vi "Secure-Release Region.vi"(7 "Action":enum16{"Secure", "Release"}(ring), 8 "error in (no error)":errorcluster, 10 "Control In":T1={"I-O.lvclass"=refnum, "Motion.lvclass"=refnum, "Dispenser.lvclass"=refnum}, 11 "Workspace in":refnum<class "Component Tray.lvclass">) -> (0 "error out":errorcluster, 2 "Control Out":T1, 3 "Workspace out":refnum<class "Component Tray.lvclass">)   [LabVIEW 2016, in "Component Tray.lvclass"]
uses:
  Component Tray.lvclass
  C:/Users/HEP Gantry/Documents/Assembly/V5/Classes/Workspace/Fixture.lvclass
  Controller/Controllers.ctl
  Controller/I-O/I-O.lvclass
  Controller/Motion/A3200/A3200.lvclass
  Controller/Dispenser/Dispenser.lvclass
  Controller/Motion/Motion.lvclass
  Fixture.lvclass/Fixture.ctl
  Read Gantry Region.vi
  Read Position.vi
  Fixture.lvclass
  Controller/Controller.lvclass
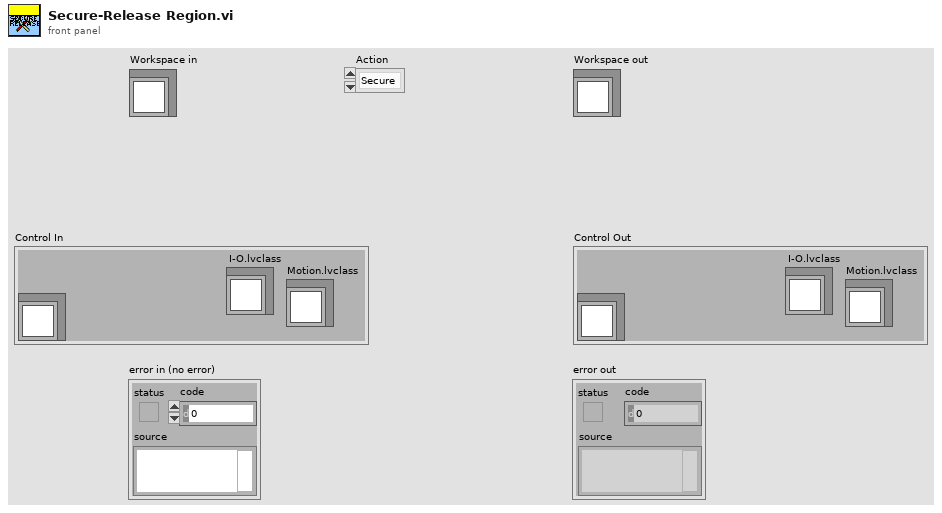
[diagram p1: front panel]
types:
  T1 = typedef "Controller.lvclass/Controllers.ctl" = cluster{"I-O.lvclass":refnum<class "I-O.lvclass">, "Motion.lvclass":refnum<class "Motion.lvclass">, "Dispenser.lvclass":refnum<class "Dispenser.lvclass">}
  T2 = typedef "I-O.lvclass/Pin Map.ctl" = cluster{"Region Valves":i32[], "Extra Valves":dbl[][], "Tool Primary Valve":i32, "Tool Secondary Valve":i32, "Region Sensors":i32[], "Extra Sensors":dbl[][], "Tool Primary Sensor":dbl, "Tool Secondary Sensor":dbl, "Compression Sensor":dbl, "5V":i32}
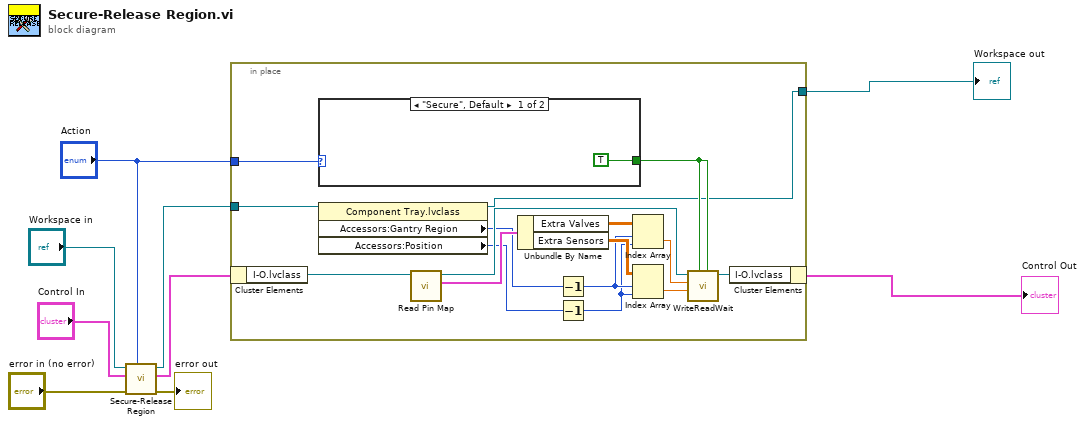
[diagram p0: block diagram]
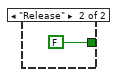
[diagram p2: hidden frame]
diagram:
  n1 = call-parent "Secure-Release Region.vi"("Action"="Action", "error in (no error)"="error in (no error)", "Control In"="Control In", "Fixture in"="Workspace in") -> ("error out"=→"error out":errorcluster, "Control Out"=w5:T1, "Fixture out"=w2:refnum<class "Component Tray.lvclass">)  [unwired: 5 in]
  n2 = in-place {
    in-place-border: "Action" -> [w22]
    in-place-border: w2 -> [w19]
    in-place-border: [w12] -> w1
    n3 = in-place-cluster #1(w5) -> ("I-O.lvclass"=w24:refnum<class "I-O.lvclass">)
    n4 = case shown="\"Secure\", Default" w22 {
      tunnel: [TRUE FALSE] -> w23
      frame "Secure", Default {
      }
      frame "Release" {
      }
    }
    n5 = property class="Component Tray.lvclass"(reference=w19) -> (reference out=w12:refnum<class "Component Tray.lvclass">, "Accessors:Gantry Region"=w16:i32, "Accessors:Position"=w14:i32)  [unwired: 1 in, 1 out]
    n6 = call-dynamic "Read Pin Map.vi"("I-O in"=w24) -> ("Pin Map"=w25:T2, "I-O out"=w21:refnum<class "I-O.lvclass">)  [unwired: 8 in, 1 out]
    n7 = Unbundle By Name(w25) -> ("Extra Valves"=w18:dbl[][], "Extra Sensors"=w17:dbl[][])
    n8 = Decrement(x=w16) -> (x-1=w15:i32)
    n9 = Decrement(x=w14) -> (x-1=w13:i32)
    n10 = Index Array(array=w18, index (row)=w15, index (col)=w13) -> (element=w11:dbl)
    n11 = Index Array(array=w17, index (row)=w15, index (col)=w13) -> (element=w10:dbl)
    n12 = call "WriteReadWait.vi"("Read Value"=w23, "Write Value"=w23, "Read"=w10, "Write"=w11, "I-O in"=w21) -> ("I-O out"=w20:refnum<class "I-O.lvclass">)  [unwired: 5 in, 1 out]
    n13 = in-place-cluster #1("I-O.lvclass"=w20) -> (→"Control Out":T1)
  }
  "Workspace out" <- w1
